vi "SaveMean_Example_IMAQ.vi"() -> ()   [LabVIEW 2019]
doc: "This example shows how to record an image sequence, get the mean of that sequence and save it to file afterwards.\nIt is a good starting point for writing own applications.\nBut it will not be fail save, i.e. doesnt react on errors, just handles them forward to the end\n\nUsage:\nSelect your required image count you want to average over before you start the program.\nOnce started, the camera class will be initialized and images will be recorded automatically.\nTWhen acquisition has finished the mean image is read and shown.\nNow you can crop the image using the ROI parameters and select a file path.\nBy clicking save, the mean image is saved with the selected file format using the current roi setting\nThis also finishes the program and will force an exit of the camera class"
uses:
  camera/Camera.lvclass
panel:
  out "rawImage":u16[][](array[numeric])
  out "Image":T1(plugin-control)
  in  "data_format":T2(ring)=enum."Mono16"
  in  "Image Index":u32 max=9
  in  "saveImages":bool
  in  "SavePath":path
  out "Recorded Images":u32
  in  "Quit":bool
  in  "cropY1":u64=2 min=2 max=1040 step=1
  in  "cropX1":u64=2 min=2 max=1392 step=1
  in  "cropY0":u64=1 min=1 max=1039 step=1
  in  "cropX0":u64=1 min=1 max=1391 step=1
  out "Image Height":u16
  out "Image Width":u16
  in  "dwImgCount":u32=10 caption="Required Number of Images" max=4023
  out "Error":errorcluster {"code" format="%x"}
  # "This example shows how to record an image sequence, get the mean of that sequence and save it to file afterwards.\nIt is a good starting point for writing own applications.\nBut it will not be fail save, i.e. doesnt react on errors, just handles them forward to the end\n\nUsage:\nSelect your required image count you want to average over before you start the program.\nOnce started, the camera class will be initialized and images will be recorded automatically.\nTWhen acquisition has finished the mean image is read and shown.\nNow you can crop the image using the crop parameters and select a file path.\nBy clicking save, the mean image is saved with the selected file format using the current roi setting\nThis also finishes the program and will force an exit of the camera class"
  # "pco.labview"
  # "Camera Setup"
  # "Recording Control"
  # "Parameters for image readout"
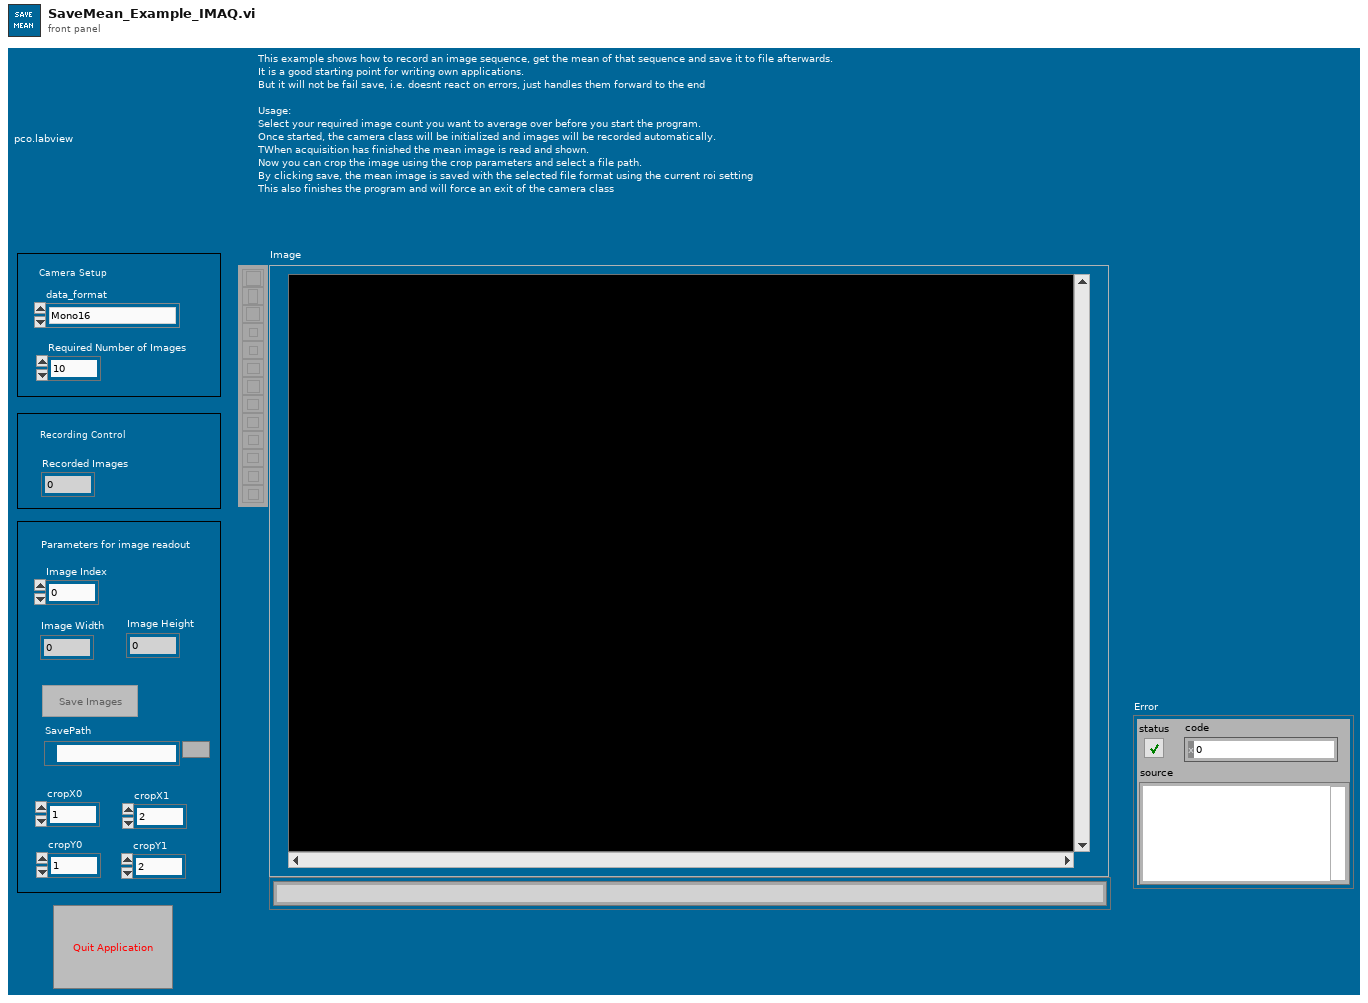
[diagram p1: front panel]
types:
  T1 = typedef "IMAQ Image.ctl" = refnum<image>
  T2 = enum16{"Undefined", "Mono8", "Mono16", "BGRA8", "RGBA8", "BGRA16", "RGBA16", "CompressedMono8"}
  T3 = enum8{"Enabled", "Disabled", "Disabled and Grayed Out"}
  T4 = enum16{"sequence", "sequence non blocking", "ring buffer", "fifo", "tif", "multitif", "pcoraw", "b16", "dicom", "multidicom", "camram_ring", "camram_segment"}
  T5 = cluster{"serial":u32, "type":u16, "sub_type":u16, "interface_type":u16, "bit_resolution":u16, "min_exposure_time_s":dbl, "max_exposure_time_s":dbl, "min_exposure_step_s":dbl, "min_delay_time_s":dbl, "max_delay_time_s":dbl, "min_delay_step_s":dbl, "min_width":u64, "min_height":u64, "max_width":u64, "max_height":u64, "roi_step_horz":u64, "roi_step_vert":u64, "roi_symmetric_horz":bool, "roi_symmetric_vert":bool, "has_timestamp_mode":bool, "has_timestamp_mode_ascii_only":bool, "pixelrate_vec":u32[], "conversion_factor_vec":sgl[], "has_trigger_mode_extexpctrl":bool, "has_acquire_mode":bool, "has_ext_acquire_mode":bool, "has_metadata_mode":bool, "has_ram":bool, "binning_horz_vec":u16[], "binning_vert_vec":u16[], "has_average_binning":bool, "pixel_format_vec":u32[]}
  T6 = typedef "Image Type" = u32
  T7 = typedef "Camera.lvclass/binning.ctl" = cluster{"vert":u16, "horz":u16, "mode":u16}
  T8 = cluster{"exposure_time_s":dbl, "delay_time_s":dbl, "roi":cluster{"x0":u64, "y0":u64, "x1":u64, "y1":u64}, "timestamp_mode":u16, "pixelrate":u32, "conversion_factor":sgl, "trigger_mode":u16, "acquire_mode":u16, "acquire_sequence_number":u32, "metadata_mode":u16, "noisefilter_mode":u16, "pixel_format":u32, "binning":T7, "auto_exposure":cluster{"region":u16, "min_exposure_s":dbl, "max_exposure_s":dbl}}
  T9 = cluster{"Plane 4 (alpha)":u16, "Plane 1 (Red)":u16, "Plane 2 (Green)":u16, "Plane 3 (Blue)":u16}[][]
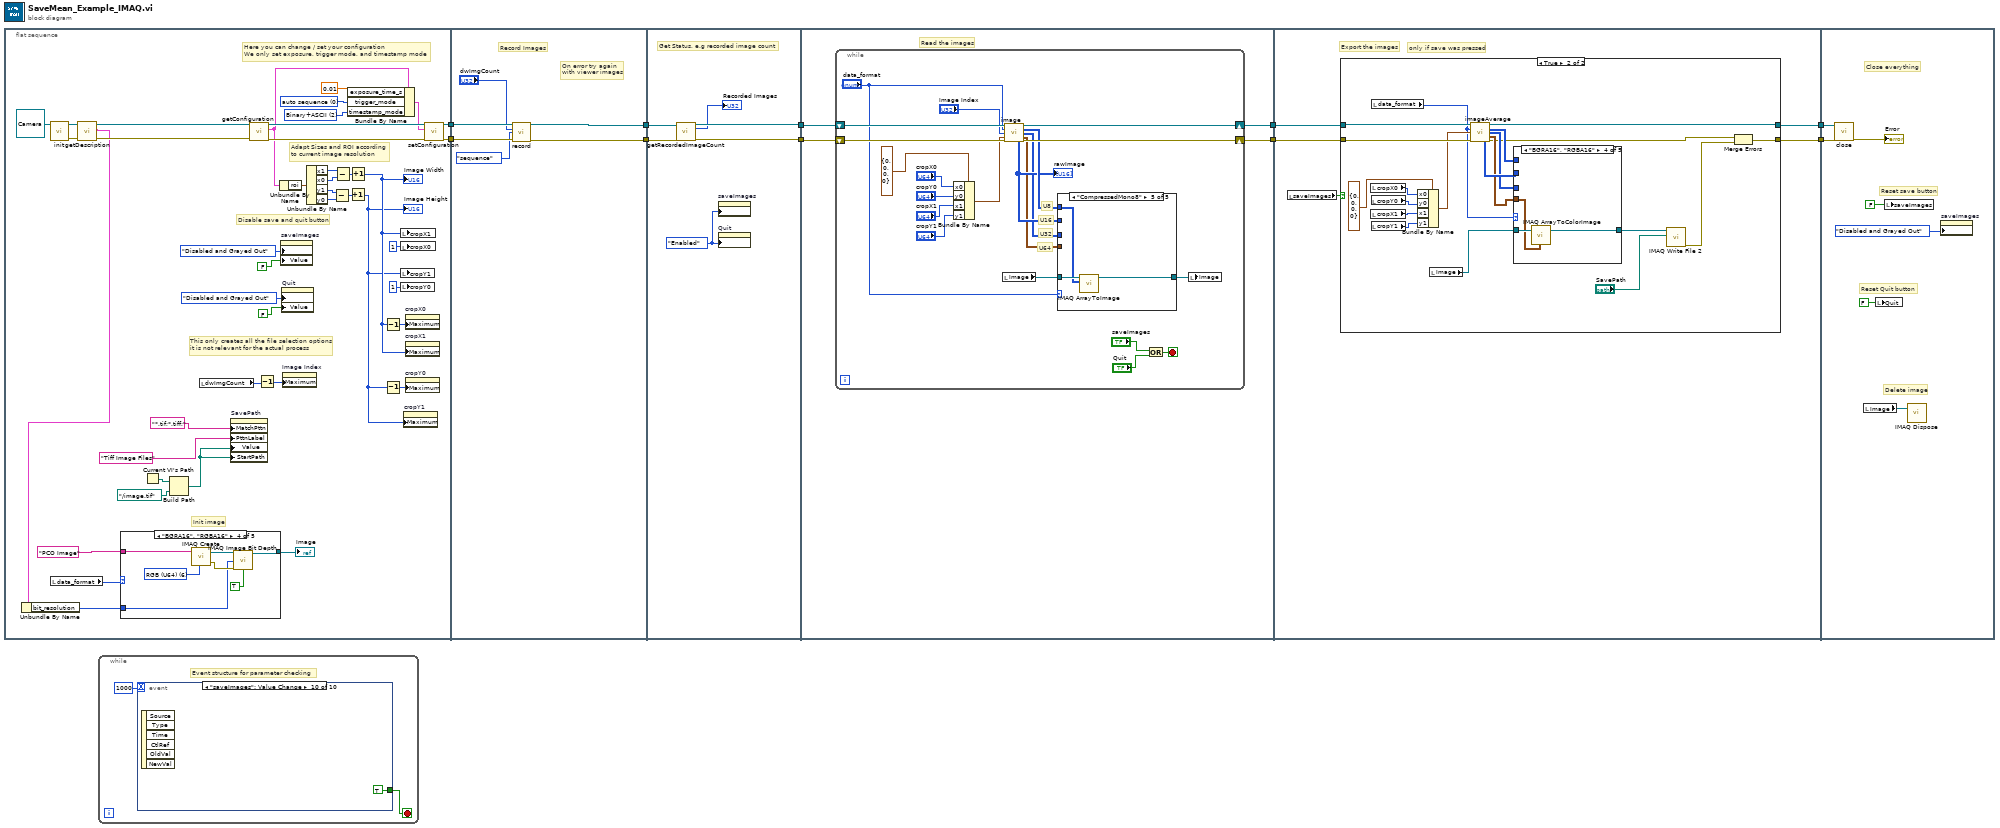
[diagram p0: block diagram]
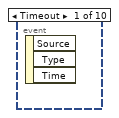
[diagram p2: hidden frame]
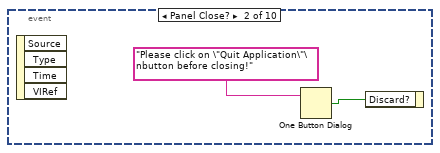
[diagram p3: hidden frame]
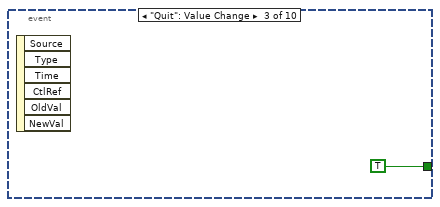
[diagram p4: hidden frame]
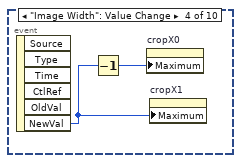
[diagram p5: hidden frame]
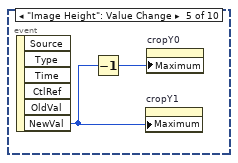
[diagram p6: hidden frame]
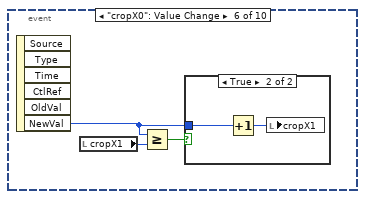
[diagram p7: hidden frame]
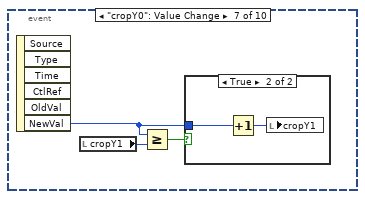
[diagram p9: hidden frame]
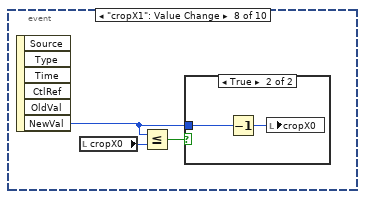
[diagram p11: hidden frame]
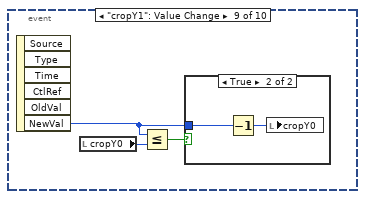
[diagram p13: hidden frame]
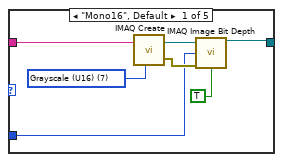
[diagram p15: hidden frame]
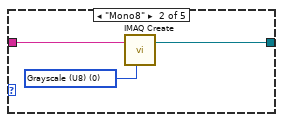
[diagram p16: hidden frame]
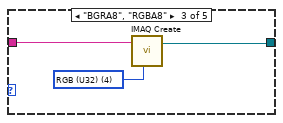
[diagram p17: hidden frame]
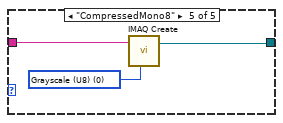
[diagram p18: hidden frame]
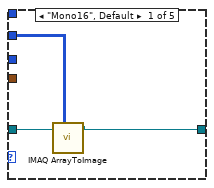
[diagram p19: hidden frame]
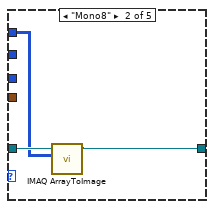
[diagram p20: hidden frame]
diagram:
  n1 = flat-sequence {
    tunnel: [w46] -> w10
    tunnel: [w45] -> w9
    tunnel: w10 -> [w82]
    tunnel: w9 -> [w81]
    tunnel: [w79] -> w8
    tunnel: [w78] -> w7
    tunnel: w8 -> [w88]
    tunnel: w7 -> [w87]
    tunnel: [w86] -> w6
    tunnel: [w85] -> w5
    tunnel: w6 -> [w91]
    tunnel: w5 -> [w92]
    tunnel: [w90] -> w4
    tunnel: [w89] -> w2
    tunnel: w4 -> [w132]
    tunnel: [w131] -> w3
    tunnel: w2 -> [w130]
    tunnel: [w129] -> w1
    tunnel: w3 -> [w177]
    tunnel: w1 -> [w176]
    frame #0 {
      w30 = u16 2 items=["OFF", "Binary", "Binary+ASCII", "ASCII"] ("TimestampMode")
      w52 = u16 0 items=["auto sequence"=0, "software trigger"=1, "external exposure start & software trigger"=2, "external exposure control"=3, "external synchronized"=4, "fast external exposure control"=5, "external CDS control"=6, "slow external exposure control"=7, "external synchronized HDSDI"=258] ("TriggerMode")
      # "Here you can change / set your configuration\nWe only set exposure, trigger mode, and timestamp mode"
      # "Init image"
      # "This only creates all the file selection options\nit is not relevant for the actual process"
      # "Adapt Sizes and ROI according\nto current image resolution"
      # "Disable save and quit button"
      n2 = call-dynamic "init.vi"("Camera in"=refnum<class "Camera.lvclass"> refnum ("PCOCamera in")) -> ("Camera out"=w16:refnum<class "Camera.lvclass">, "error out"=w17:errorcluster)  [unwired: 8 in]
      n3 = local read "data_format"() -> (w20:T2)
      n4 = call-dynamic "getDescription.vi"("error in (no error)"=w17, "Camera in"=w16) -> ("error out"=w14:errorcluster, "description"=w13:T5, "Camera out"=w15:refnum<class "Camera.lvclass">)  [unwired: 7 in]
      n5 = Unbundle By Name(w13) -> ("bit_resolution"=w12:u16)
      n6 = case shown="\"BGRA16\", \"RGBA16\"" w20 {
        tunnel: "PCO Image" ("Image Name") -> [w59 w63 w65 w72 w75]
        tunnel: [w55 w61 w64 w69 w74] -> w19
        tunnel: w12 -> [w54 _ _ w67 _]
        frame "Mono16", Default {
          w60 = T6 7 items=["Grayscale (U8)", "Grayscale (I16)", "Grayscale (SGL)", "Complex (CSG)", "RGB (U32)", "HSL (U32)", "RGB (U64)", "Grayscale (U16)"] ("Image Type")
          n7 = call "IMAQ Create"("Image Name"=w59, "Image Type"=w60) -> ("New Image"=w57:T1, "error out"=w56:errorcluster)  [unwired: 3 in]
          n8 = call "IMAQ Image Bit Depth"("Image"=w57, "Bit Depth (0)"=w54, "error in (no error)"=w56, "Get/Set Bit Depth? (Set)"=TRUE) -> ("Image Out"=w55:T1)  [unwired: 9 in, 2 out]
        }
        frame "Mono8" {
          w62 = T6 0 items=["Grayscale (U8)", "Grayscale (I16)", "Grayscale (SGL)", "Complex (CSG)", "RGB (U32)", "HSL (U32)", "RGB (U64)", "Grayscale (U16)"] ("Image Type")
          n9 = call "IMAQ Create"("Image Name"=w63, "Image Type"=w62) -> ("New Image"=w61:T1)  [unwired: 3 in, 1 out]
        }
        frame "BGRA8", "RGBA8" {
          w66 = T6 4 items=["Grayscale (U8)", "Grayscale (I16)", "Grayscale (SGL)", "Complex (CSG)", "RGB (U32)", "HSL (U32)", "RGB (U64)", "Grayscale (U16)"] ("Image Type")
          n10 = call "IMAQ Create"("Image Name"=w65, "Image Type"=w66) -> ("New Image"=w64:T1)  [unwired: 3 in, 1 out]
        }
        frame "BGRA16", "RGBA16" {
          w73 = T6 6 items=["Grayscale (U8)", "Grayscale (I16)", "Grayscale (SGL)", "Complex (CSG)", "RGB (U32)", "HSL (U32)", "RGB (U64)", "Grayscale (U16)"] ("Image Type")
          n11 = call "IMAQ Create"("Image Name"=w72, "Image Type"=w73) -> ("New Image"=w70:T1, "error out"=w68:errorcluster)  [unwired: 3 in]
          n12 = call "IMAQ Image Bit Depth"("Image"=w70, "Bit Depth (0)"=w67, "error in (no error)"=w68, "Get/Set Bit Depth? (Set)"=TRUE) -> ("Image Out"=w69:T1)  [unwired: 9 in, 2 out]
        }
        frame "CompressedMono8" {
          w76 = T6 0 items=["Grayscale (U8)", "Grayscale (I16)", "Grayscale (SGL)", "Complex (CSG)", "RGB (U32)", "HSL (U32)", "RGB (U64)", "Grayscale (U16)"] ("Image Type")
          n13 = call "IMAQ Create"("Image Name"=w75, "Image Type"=w76) -> ("New Image"=w74:T1)  [unwired: 3 in, 1 out]
        }
      }
      "Image" <- w19
      n14 = Current VI's Path() -> (path=w27:path)
      n15 = Build Path(base path=w27, name or relative path=path "../image.tif" ("SavePath")) -> (appended path=w24:path)
      n16 = local read "dwImgCount"() -> (w22:u32)
      n17 = property on="SavePath" class="Path"("MatchPttn"="*.tif;*.tiff;" ("pattern (all files)"), "PttnLabel"="Tiff Image Files" ("pattern label"), "Value"=w24, "StartPath"=w24) -> ()  [unwired: 2 in, 2 out]
      n18 = call-dynamic "getConfiguration.vi"("error in (no error)"=w14, "Camera in"=w15) -> ("error out"=w50:errorcluster, "configuration"=w40:T8, "Camera out"=w51:refnum<class "Camera.lvclass">)  [unwired: 7 in]
      n19 = Decrement(x=w22) -> (x-1=w23:u32)
      n20 = Unbundle By Name(w40) -> ("roi"=w39:cluster{"x0":u64, "y0":u64, "x1":u64, "y1":u64})
      n21 = property on="saveImages" class="Bool (strict)"("DisabledEnum"=T3."Disabled and Grayed Out" ("Disabled"), "Value"=FALSE ("Stop")) -> ()  [unwired: 2 in, 2 out]
      n22 = property on="Quit" class="Bool (strict)"("DisabledEnum"=T3."Disabled and Grayed Out" ("Disabled"), "Value"=FALSE ("Stop")) -> ()  [unwired: 2 in, 2 out]
      n23 = property on="Image Index" class="DigNum (strict)"("Maximum"=w23) -> ()  [unwired: 2 in, 2 out]
      n24 = Unbundle By Name(w39) -> ("x1"=w37:u64, "x0"=w38:u64, "y1"=w35:u64, "y0"=w36:u64)
      n25 = Subtract(x=w35, y=w36) -> (x-y=w33:u64)
      n26 = Subtract(x=w37, y=w38) -> (x-y=w34:u64)
      n27 = Bundle By Name(cluster=w40, "exposure_time_s"=0.01, "trigger_mode"=w52, "timestamp_mode"=w30) -> (w49:T8)
      n28 = Increment(x=w33) -> (x+1=w31:u64)
      "Image Height" <- w31
      n29 = Increment(x=w34) -> (x+1=w32:u64)
      "Image Width" <- w32
      n30 = Decrement(x=w32) -> (x-1=w42:u64)
      n31 = Decrement(x=w31) -> (x-1=w41:u64)
      n32 = local write "cropX1"(w32) -> ()
      n33 = local write "cropX0"(u16 1 ("roiY0")) -> ()
      n34 = local write "cropY1"(w31) -> ()
      n35 = local write "cropY0"(u16 1 ("roiY0")) -> ()
      n36 = property on="cropY1" class="DigNum (strict)"("Maximum"=w31) -> ()  [unwired: 2 in, 2 out]
      n37 = property on="cropX0" class="DigNum (strict)"("Maximum"=w42) -> ()  [unwired: 2 in, 2 out]
      n38 = property on="cropX1" class="DigNum (strict)"("Maximum"=w32) -> ()  [unwired: 2 in, 2 out]
      n39 = property on="cropY0" class="DigNum (strict)"("Maximum"=w41) -> ()  [unwired: 2 in, 2 out]
      n40 = call-dynamic "setConfiguration.vi"("error in (no error)"=w50, "configuration"=w49, "Camera in"=w51) -> ("error out"=w45:errorcluster, "Camera out"=w46:refnum<class "Camera.lvclass">)  [unwired: 7 in]
    }
    frame #1 {
      # "On error try again \nwith viewer images"
      # "Record Images"
      n41 = call-dynamic "record.vi"("Camera in"=w82, "num_images"="dwImgCount", "record_mode"=T4."sequence", "error in (no error)"=w81) -> ("Camera out"=w79:refnum<class "Camera.lvclass">, "error out"=w78:errorcluster)  [unwired: 10 in]
    }
    frame #2 {
      w83 = T3."Enabled" ("Disabled")
      # "Get Status, e.g recorded image count"
      n42 = call-dynamic "getRecordedImageCount.vi"("Camera in"=w88, "error in (no error)"=w87) -> ("Camera out"=w86:refnum<class "Camera.lvclass">, "recorded_image_count"=→"Recorded Images":u32, "error out"=w85:errorcluster)  [unwired: 11 in]
      n43 = property on="saveImages" class="Bool (strict)"("DisabledEnum"=w83) -> ()  [unwired: 2 in, 2 out]
      n44 = property on="Quit" class="Bool (strict)"("DisabledEnum"=w83) -> ()  [unwired: 2 in, 2 out]
    }
    frame #3 {
      # "Read the images"
      n45 = while {
        shift-right: [w111] -> w90
        shift-left: w91 -> [w113]
        shift-right: [w106] -> w89
        shift-left: w92 -> [w112]
        stop <- w104 stop-if-true
        # "U64"
        # "U32"
        # "U16"
        # "U8"
        n46 = Bundle By Name(cluster=cluster{"x0":u64, "y0":u64, "x1":u64, "y1":u64} {"x0"=0, "y0"=0, "x1"=0, "y1"=0} ("roi"), "x0"="cropX0", "y0"="cropY0", "x1"="cropX1", "y1"="cropY1") -> (w102:cluster{"x0":u64, "y0":u64, "x1":u64, "y1":u64})
        n47 = local read "Image"() -> (w95:T1)
        n48 = call-dynamic "image.vi"("Camera in"=w113, "data_format"="data_format", "image_index"="Image Index", "crop"=w102, "error in (no error)"=w112) -> ("Camera out"=w111:refnum<class "Camera.lvclass">, "image (U8)"=w99:u8[][], "image (U32)"=w97:u32[][], "image (U64)"=w96:T9, "raw_image (U16)"=w98:u16[][], "error out"=w106:errorcluster)  [unwired: 2 in, 3 out]
        "rawImage" <- w98
        n49 = case shown="\"CompressedMono8\"" "data_format" {
          tunnel: w95 -> [w116 w119 w122 w125 w128]
          tunnel: [w114 w117 w121 w123 w127] -> w94
          tunnel: w96 -> [_ _ _ w124 _]
          tunnel: w97 -> [_ _ w120 _ _]
          tunnel: w99 -> [_ w118 _ _ w126]
          tunnel: w98 -> [w115 _ _ _ _]
          frame "Mono16", Default {
            n50 = call "IMAQ ArrayToImage"("Image Pixels (U16)"=w115, "Image"=w116) -> ("Image Out"=w114:T1)  [unwired: 8 in, 1 out]
          }
          frame "Mono8" {
            n51 = call "IMAQ ArrayToImage"("Image Pixels (U8)"=w118, "Image"=w119) -> ("Image Out"=w117:T1)  [unwired: 8 in, 1 out]
          }
          frame "BGRA8", "RGBA8" {
            n52 = call "IMAQ ArrayToColorImage"("Image Pixels (U32)"=w120, "Image"=w122) -> ("Image Out"=w121:T1)  [unwired: 3 in, 1 out]
          }
          frame "BGRA16", "RGBA16" {
            n53 = call "IMAQ ArrayToColorImage"("Image"=w125, "Image Pixels (U64)"=w124) -> ("Image Out"=w123:T1)  [unwired: 3 in, 1 out]
          }
          frame "CompressedMono8" {
            n54 = call "IMAQ ArrayToImage"("Image Pixels (U8)"=w126, "Image"=w128) -> ("Image Out"=w127:T1)  [unwired: 8 in, 1 out]
          }
        }
        n55 = Or(x="saveImages", y="Quit") -> (x .or. y?=w104:bool)
        n56 = local write "Image"(w94) -> ()
      }
    }
    frame #4 {
      # "only if save was pressed"
      # "Export the images"
      n57 = local read "saveImages"() -> (w133:bool)
      n58 = case shown="True" w133 {
        tunnel: w132 -> [w135 w154]
        tunnel: [w135 w143] -> w131
        tunnel: w130 -> [w134 w155]
        tunnel: [w134 w141] -> w129
        frame False {
        }
        frame True {
          n59 = local read "cropX0"() -> (w152:u64)
          n60 = local read "cropX1"() -> (w150:u64)
          n61 = local read "cropY0"() -> (w151:u64)
          n62 = local read "cropY1"() -> (w149:u64)
          n63 = local read "data_format"() -> (w139:T2)
          n64 = Bundle By Name(cluster=cluster{"x0":u64, "y0":u64, "x1":u64, "y1":u64} {"x0"=0, "y0"=0, "x1"=0, "y1"=0} ("roi"), "x0"=w152, "y0"=w151, "x1"=w150, "y1"=w149) -> (w148:cluster{"x0":u64, "y0":u64, "x1":u64, "y1":u64})
          n65 = local read "Image"() -> (w140:T1)
          n66 = call-dynamic "imageAverage.vi"("Camera in"=w154, "data_format"=w139, "crop"=w148, "error in (no error)"=w155) -> ("Camera out"=w143:refnum<class "Camera.lvclass">, "image (U8)"=w147:u8[][], "image (U32)"=w145:u32[][], "image (U64)"=w144:T9, "raw_image (U16)"=w146:u16[][], "error out"=w142:errorcluster)  [unwired: 5 in, 1 out]
          n67 = case shown="\"BGRA16\", \"RGBA16\"" w139 {
            tunnel: w140 -> [w158 w161 w164 w167 w170]
            tunnel: [w156 w159 w163 w165 w169] -> w137
            tunnel: w144 -> [_ _ _ w166 _]
            tunnel: w145 -> [_ _ w162 _ _]
            tunnel: w147 -> [_ w160 _ _ w168]
            tunnel: w146 -> [w157 _ _ _ _]
            frame "Mono16", Default {
              n68 = call "IMAQ ArrayToImage"("Image Pixels (U16)"=w157, "Image"=w158) -> ("Image Out"=w156:T1)  [unwired: 8 in, 1 out]
            }
            frame "Mono8" {
              n69 = call "IMAQ ArrayToImage"("Image Pixels (U8)"=w160, "Image"=w161) -> ("Image Out"=w159:T1)  [unwired: 8 in, 1 out]
            }
            frame "BGRA8", "RGBA8" {
              n70 = call "IMAQ ArrayToColorImage"("Image Pixels (U32)"=w162, "Image"=w164) -> ("Image Out"=w163:T1)  [unwired: 3 in, 1 out]
            }
            frame "BGRA16", "RGBA16" {
              n71 = call "IMAQ ArrayToColorImage"("Image"=w167, "Image Pixels (U64)"=w166) -> ("Image Out"=w165:T1)  [unwired: 3 in, 1 out]
            }
            frame "CompressedMono8" {
              n72 = call "IMAQ ArrayToImage"("Image Pixels (U8)"=w168, "Image"=w170) -> ("Image Out"=w169:T1)  [unwired: 8 in, 1 out]
            }
          }
          n73 = call-poly "IMAQ Write File 2"("File Path"="SavePath", "Image"=w137) -> ("error out"=w138:errorcluster)  [unwired: 8 in, 1 out]
          n74 = Merge Errors(w142, w138) -> (w141:errorcluster)
        }
      }
    }
    frame #5 {
      # "Delete image"
      # "Reset Quit button"
      # "Close everything"
      # "Reset save button"
      n75 = call-dynamic "close.vi"("error in (no error)"=w176, "Camera in"=w177) -> ("error out"=→"Error":errorcluster)  [unwired: 9 in]
      n76 = local read "Image"() -> (w171:T1)
      n77 = local write "Quit"(FALSE ("Stop")) -> ()
      n78 = local write "saveImages"(FALSE ("Stop")) -> ()
      n79 = call "IMAQ Dispose"("Image"=w171) -> ()  [unwired: 5 in, 1 out]
      n80 = property on="saveImages" class="Bool (strict)"("DisabledEnum"=T3."Disabled and Grayed Out" ("Disabled")) -> ()  [unwired: 2 in, 2 out]
    }
  }
  n81 = while {
    stop <- w178 stop-if-true
    # "Event structure for parameter checking"
    n82 = event shown="[9] \"saveImages\": Value Change" {
      selector: _ -> [_ _ _ _ _ _ _ _ _ _]
      dyn-events: _ -> [_ _ _ _ _ _ _ _ _ _]
      timeout: 1000 -> [_ _ _ _ _ _ _ _ _ _]
      tunnel: [_ _ TRUE _ _ _ _ _ _ TRUE] -> w178
      event Timeout {
        n83 = event-data() -> ()  [unwired: 1 in, 3 out]
      }
      event Panel Close? {
        n84 = event-data() -> ()  [unwired: 1 in, 4 out]
        n85 = One Button Dialog(message="Please click on \"Quit Application\"\nbutton before closing!") -> (true=w180:bool)  [unwired: 1 in]
        n86 = event-data("Discard?"=w180) -> ()  [unwired: 1 in, 1 out]
      }
      event "Quit": Value Change {
        n87 = event-data() -> ()  [unwired: 1 in, 6 out]
      }
      event "Image Width": Value Change {
        n88 = event-data() -> ("NewVal"=w183:u16)  [unwired: 1 in, 5 out]
        n89 = Decrement(x=w183) -> (x-1=w184:u16)
        n90 = property on="cropX0" class="DigNum (strict)"("Maximum"=w184) -> ()  [unwired: 2 in, 2 out]
        n91 = property on="cropX1" class="DigNum (strict)"("Maximum"=w183) -> ()  [unwired: 2 in, 2 out]
      }
      event "Image Height": Value Change {
        n92 = event-data() -> ("NewVal"=w185:u16)  [unwired: 1 in, 5 out]
        n93 = Decrement(x=w185) -> (x-1=w186:u16)
        n94 = property on="cropY1" class="DigNum (strict)"("Maximum"=w185) -> ()  [unwired: 2 in, 2 out]
        n95 = property on="cropY0" class="DigNum (strict)"("Maximum"=w186) -> ()  [unwired: 2 in, 2 out]
      }
      event "cropX0": Value Change {
        n96 = event-data() -> ("NewVal"=w187:u64)  [unwired: 1 in, 5 out]
        n97 = local read "cropX1"() -> (w189:u64)
        n98 = Greater Or Equal?(x=w187, y=w189) -> (x >= y?=w188:bool)
        n99 = case shown="True" w188 {
          tunnel: w187 -> [_ w191]
          frame False {
          }
          frame True {
            n100 = Increment(x=w191) -> (x+1=w190:u64)
            n101 = local write "cropX1"(w190) -> ()
          }
        }
      }
      event "cropY0": Value Change {
        n102 = event-data() -> ("NewVal"=w192:u64)  [unwired: 1 in, 5 out]
        n103 = local read "cropY1"() -> (w194:u64)
        n104 = Greater Or Equal?(x=w192, y=w194) -> (x >= y?=w193:bool)
        n105 = case shown="True" w193 {
          tunnel: w192 -> [_ w196]
          frame False {
          }
          frame True {
            n106 = Increment(x=w196) -> (x+1=w195:u64)
            n107 = local write "cropY1"(w195) -> ()
          }
        }
      }
      event "cropX1": Value Change {
        n108 = event-data() -> ("NewVal"=w197:u64)  [unwired: 1 in, 5 out]
        n109 = local read "cropX0"() -> (w199:u64)
        n110 = Less Or Equal?(x=w197, y=w199) -> (x <= y?=w198:bool)
        n111 = case shown="True" w198 {
          tunnel: w197 -> [_ w201]
          frame False {
          }
          frame True {
            n112 = Decrement(x=w201) -> (x-1=w200:u64)
            n113 = local write "cropX0"(w200) -> ()
          }
        }
      }
      event "cropY1": Value Change {
        n114 = event-data() -> ("NewVal"=w202:u64)  [unwired: 1 in, 5 out]
        n115 = local read "cropY0"() -> (w204:u64)
        n116 = Less Or Equal?(x=w202, y=w204) -> (x <= y?=w203:bool)
        n117 = case shown="True" w203 {
          tunnel: w202 -> [_ w206]
          frame False {
          }
          frame True {
            n118 = Decrement(x=w206) -> (x-1=w205:u64)
            n119 = local write "cropY0"(w205) -> ()
          }
        }
      }
      event "saveImages": Value Change {
        n120 = event-data() -> ()  [unwired: 1 in, 6 out]
      }
    }
  }
